vi "FMA1600A Build Commands.vi"(8 "Error In":errorcluster, 9 "Gas Type":T2, 10 "Unit ID":string, 11 "FMA1600A Commands":T1) -> (0 "Error Out":errorcluster, 3 "Command Output":string)   [LabVIEW 2019]
uses:
  Type Definitions/FMA1600A Gas Type.ctl
  Type Definitions/FMA1600A Commands.ctl
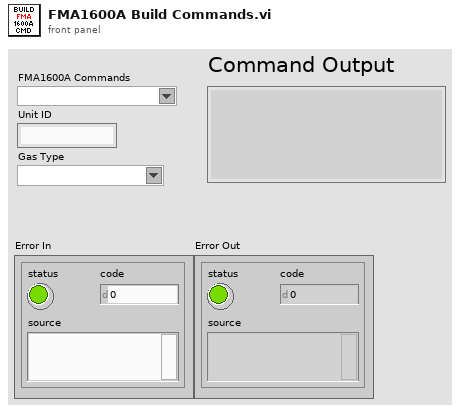
[diagram p1: front panel]
types:
  T1 = typedef "FMA1600A Commands.ctl" = string
  T2 = typedef "FMA1600A Gas Type.ctl" = string
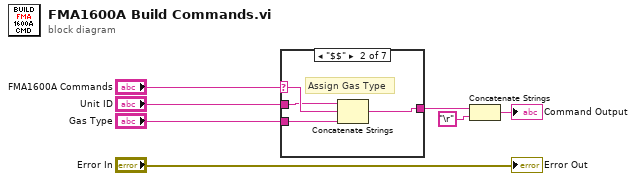
[diagram p0: block diagram]
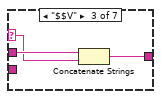
[diagram p3: hidden frame]
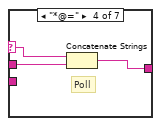
[diagram p4: hidden frame]
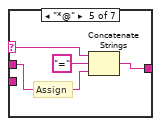
[diagram p5: hidden frame]
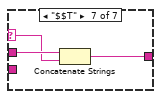
[diagram p7: hidden frame]
diagram:
  n1 = case shown="\"$$\"" "FMA1600A Commands" {
    selector: "FMA1600A Commands" -> [w8 w12 w14 w18 w22 _ w25]
    tunnel: [w8 w11 w13 w16 w19 w23 w24] -> w4
    tunnel: "Gas Type" -> [_ w10 _ _ _ w23 _]
    tunnel: "Unit ID" -> [_ w9 w15 w17 w20 _ w26]
    frame Default {
      # "Stream"
    }
    frame "$$" {
      # "Assign Gas Type"
      n2 = Concatenate Strings(w9, w12, w10) -> (w11:string)
    }
    frame "$$V" {
      n3 = Concatenate Strings(w15, w14) -> (w13:string)
    }
    frame "*@=" {
      # "Poll"
      n4 = Concatenate Strings(w18, w17) -> (w16:string)
    }
    frame "*@" {
      # "Assign"
      n5 = Concatenate Strings(w22, "=" ("string"), w20) -> (w19:string)
    }
    frame "-" {
    }
    frame "$$T" {
      n6 = Concatenate Strings(w26, w25) -> (w24:string)
    }
  }
  n7 = Concatenate Strings(w4, "\r") -> (→"Command Output":string)
  "Error Out" <- "Error In"
